vi "Com Errori.vi"(0 "VISA session":refnum<visa-resource-name>, 3 "Errori in":i64, 6 "Max Errori":i64, 7 "error in (no error)":errorcluster) -> (20 "dup VISA session":refnum<visa-resource-name>, 23 "Errori out":i64, 26 "Chiudi com":bool, 27 "error out":errorcluster)   [LabVIEW 2019]
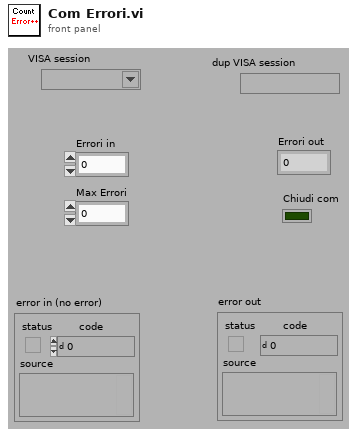
[diagram p1: front panel]
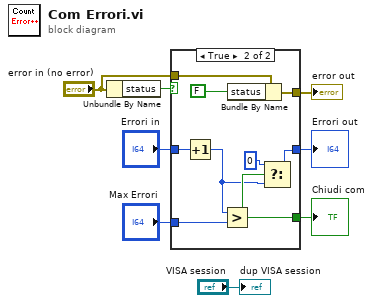
[diagram p0: block diagram]
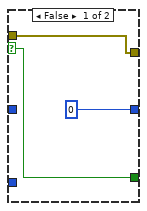
[diagram p2: hidden frame]
diagram:
  n1 = Unbundle By Name("error in (no error)") -> ("status"=w7:bool)
  n2 = case shown="True" w7 {
    selector: w7 -> [w10 _]
    tunnel: "Errori in" -> [_ w20]
    tunnel: [0 w14] -> w5
    tunnel: "Max Errori" -> [_ w19]
    tunnel: [w10 w15] -> w3
    tunnel: "error in (no error)" -> [w9 w18]
    tunnel: [w9 w17] -> w1
    frame False {
    }
    frame True {
      n3 = Increment(x=w20) -> (x+1=w12:i64)
      n4 = Greater?(x=w12, y=w19) -> (0:w15:bool)
      n5 = Bundle By Name(cluster=w18, "status"=FALSE) -> (w17:errorcluster)
      n6 = Select(t=0, s=w15, f=w12) -> (s? t:f=w14:i64)
    }
  }
  "error out" <- w1
  "Errori out" <- w5
  "Chiudi com" <- w3
  "dup VISA session" <- "VISA session"
